vi "File Conversion.vi"(1 "Initial File Path":path) -> ()   [LabVIEW 2018]
uses:
  <vilib>/regexp/Match Regular Expression.xnode
panel:
  out "whole match":string
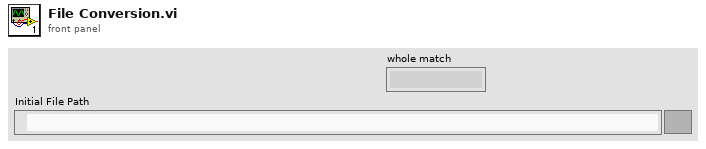
[diagram p1: front panel]
types:
  T1 = enum16{"open", "open or create", "create or replace", "create", "open (read-only)"}
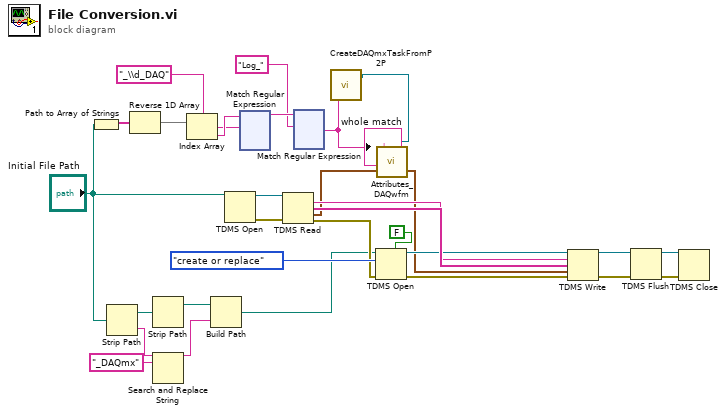
[diagram p0: block diagram]
diagram:
  n1 = Path to Array of Strings(0:"Initial File Path") -> (2:w8:string[])  [unwired: 1 out]
  n2 = Strip Path(path="Initial File Path") -> (stripped path=w15:path, name=w12:string)
  n3 = Reverse 1D Array(array=w8) -> (reversed array=w7:string[])
  n4 = Strip Path(path=w15) -> (stripped path=w14:path)  [unwired: 1 out]
  n5 = Search and Replace String(input string=w12, search string="_DAQmx") -> (result string=w10:string)  [unwired: 6 in, 3 out]
  n6 = Index Array(array=w7) -> (element=w6:string)  [unwired: 1 in]
  n7 = Build Path(base path=w14, name or relative path=w10) -> (appended path=w13:path)
  n8 = TDMS Open(11:"Initial File Path") -> (0:w18:errorcluster, 3:w17:refnum<k34>)  [unwired: 6 in]
  n9 = xnode "Match Regular Expression"("input string"=w6, "regular expression"="_\\d_DAQ") -> ("before match"=w4:string)  [unwired: 4 in, 4 out]
  n10 = TDMS Read(0:w17, 11:w18) -> (6:w25:string, 8:w26:string[], 10:w20:waveform(dbl)[], 15:w16:errorcluster)  [unwired: 6 in, 2 out]
  n11 = xnode "Match Regular Expression"("input string"=w4, "regular expression"="Log_") -> ("after match"=w1:string)  [unwired: 4 in, 4 out]
  "whole match" <- w1
  n12 = call "CreateDAQmxTaskFromP2P.vi"("DAQmx Device Name"=w1) -> ("task out"=w2:refnum<k21>)  [unwired: 1 out]
  n13 = TDMS Open(5:FALSE ("create index file? (T)"), 8:w16, 10:T1."create or replace" ("operation (0:open)"), 11:w13) -> (0:w24:errorcluster, 3:w23:refnum<k34>)  [unwired: 3 in]
  n14 = call "Attributes_DAQwfm.vi"("data"=w20, "Refnum in"=w2) -> ("Array"=w19:waveform(dbl)[])  [unwired: 1 out]
  n15 = TDMS Write(0:w23, 5:w25, 7:w26, 9:w19, 11:w24) -> (4:w29:refnum<k34>, 15:w30:errorcluster)  [unwired: 1 in, 2 out]
  n16 = TDMS Flush(4:w30, 7:w29) -> (0:w27:errorcluster, 3:w28:refnum<k34>)
  n17 = TDMS Close(8:w27, 11:w28) -> ()  [unwired: 2 out]
